vi "BeeperCAL2014.VI"(0 "offset":dbl=137.0, 1 "Init":bool=TRUE, 2 "sample rate":dbl=48000.0, 3 "number of samples":i32=512, 4 "Upper Cut-Off":dbl=4000.0, 5 "Lower Cut-Off":dbl=2000.0, 7 "error in":errorcluster, 19 "Serial":string) -> (10 "N Harmonics":i32, 12 "Harmonic Array":T1(array[cluster]), 13 "error out":errorcluster, 14 "PASS/FAIL 4":bool caption="PASS/FAIL", 15 "fundamental frequency":dbl format="%.2p", 16 "fundamental amplitude":dbl, 17 "fundamental dB output":dbl, 18 "THD":dbl format="%.2p")   [LabVIEW 2014]
uses:
  <vilib>/express/express analysis/Spectral/Block/exnSpectralBlock spectral measurements peak poly.vi
  <vilib>/express/express analysis/Spectral/Block/exnSpectralBlock spectral measurements peak WFM.vi
  <vilib>/measure/matone.llb/Extract Multiple Tone Information 1 Chan.vi
  <vilib>/measure/matone.llb/Harmonic Distortion Analyzer 1 Chan.vi
  <vilib>/express/express analysis/Spectral/XNode/ExpressSpectralMeasurementsBlockNode.xnode
  <vilib>/measure/NI_MAPro.lvlib
panel:
  out "Beeper Time Domain AC":waveform(dbl)(graph)={"t0"=timestamp(0.0010416666666666667 s since 1904-01-01), "dt"=2.0833333333333333e-05, "Y"=array[205 elements], "attributes"=variant("NI_ChannelName"=variant(string "Filtered (Extracted)"), "NI_ExpIsRelativeTime"=variant(bool TRUE), "NI_ExpStartTimeStamp"=variant(timestamp timestamp(3490807910.470092 s since 1904-01-01)), "NI_ExpTimeStamp"=variant(timestamp timestamp(3490807910.4711337 s since 1904-01-01)), "NI_ExpXDimension"=variant(string "t"), "NI_OriginalChannelName"=variant(string "Filtered"))}
  out "FFT Mask":dynamicdata(graph)=[{"t0"=timestamp(0 s since 1904-01-01), "dt"=160.53511884163183, "Y"=[0.01862930946391062, 0.031426642217661484, 0.028979598239673703, 0.024709926366084507, 0.012017232364681342, 0.011717656169097746, 0.011122701775221618, 0.001466420910336564, 0.007559244860713749, 0.009360343024873896, 0.003456556665288603, 0.0067897156296726074, 0.006203684074720098, 0.00631879509417875, 0.012993104805963341, 0.013327012696816912, 0.0356049653294887, 0.2818839469028935, 1.2722755465923246, 1.198586262791819, 0.2096225801168994, 0.03758360783596433, 0.010470687908423763, 0.0044974648911843005, 0.004067655995640319, 0.0012643427161311317, 0.0018238117756748699, 0.003084844757409455, 0.00168924041789103, 0.0034902948133270135, 0.0018217384819525847, 0.00188115142234715, 0.0013349862994453566, 0.0012364116957955678, 0.0009009915470407127, 0.0016168191099444537, 0.003914549671586599, 0.007639197093317019, 0.0025429875562595315, 0.0008863144299645895, 0.000625970666921518, 0.00012529417135776933, 0.00022916937706817103, 8.05943746999969e-05, 0.0002947428004910281, 0.0002087071302997354, 0.00040486818402033474, 0.0003375545596782854, 0.0002959939659886654, 0.0002699299152619309, 0.00013911678768285866, 4.346861415304848e-05, 0.0001340626371251187, 0.00016265618612929948, 0.0001476836700813654, 0.00039981352334013366, 0.00035508436857194415, 6.626140200756173e-05, 3.88995080941158e-05, 3.119123025937372e-05, 2.5285638387376754e-05, 4.886844544186635e-05, 7.271737186606323e-05, 5.3880406295179994e-05, 1.0072539300096652e-05, 2.3422235573147303e-05, 3.2314657446449763e-06, 1.6990206739975872e-05, 1.134108398471203e-05, 4.178417309496945e-06, 1.0252243489860926e-05, 9.766164633672498e-06, 1.3132869053438505e-05, 1.527288254858445e-05, 3.3272188602078897e-05, 1.2771336225145865e-05, 4.473167784884164e-06, 4.620966317927218e-06, 5.8214805857980874e-06, 2.379626005199326e-06, 2.9329660287990012e-06, 1.3631432808303542e-06, 3.4991665124997253e-06, 1.0655970567577459e-06, 4.419526022999793e-07, 2.1382029521115426e-06, 1.475862427158877e-07, 1.9584391227532084e-06, 2.0860245880026544e-06, 2.129493795041458e-06, 1.121334519682653e-06, 2.872638431024709e-06, 1.8550832235640507e-06, 1.4625248451505506e-06, 5.315345648632081e-07, 8.534708408493283e-07, 3.283129119564777e-07, 5.02807829864226e-07, 2.4382890249089887e-07, 6.188312885710458e-07, 5.081982604412368e-07, 2.1608286873766714e-07, 4.989348320620008e-07, 4.019887501348107e-07, 2.6797818414105616e-07, 4.4343144544713926e-07, 2.739673611594064e-07, 3.601606569482968e-07, 2.4474532583807605e-07, 2.836248881840115e-07, 3.176917348943672e-07, 2.1349864844518757e-07, 2.92082878448765e-07, 2.214756065002239e-07, 2.8606260405775217e-07, 1.8201583112405534e-07, 2.4372776748657747e-07, 2.028220893859686e-07, 2.0375064159335707e-07, 2.1300679020045898e-07, 1.7890992742712778e-07, 1.8547111735493437e-07, 1.7611449860683832e-07, 1.7875609596142585e-07, 1.6297443335424254e-07, 1.589828987944283e-07, 1.5841649477268463e-07, 1.456025867482396e-07, 1.4721535218519734e-07, 1.383699844195478e-07, 1.3710525723389903e-07, 1.305385615924326e-07, 1.2606070999131247e-07, 1.227773533123688e-07, 1.1920861575851639e-07, 1.1531047964591549e-07, 1.1224234459715743e-07, 1.0871712177752873e-07, 1.0589636424703531e-07, 1.031615300858949e-07, 1.0068840478885112e-07, 9.833545832303213e-08, 9.629379899415174e-08, 9.448219109599016e-08, 9.29052890739438e-08, 9.158747866699481e-08, 9.052317514966884e-08, 8.972112518164855e-08, 8.918448214399814e-08, 8.891552686030246e-08]}, {"t0"=timestamp(0 s since 1904-01-01), "dt"=160.53511884163183, "Y"=[nan, nan, nan, nan, nan, nan, nan, nan, nan, nan, nan, nan, nan, nan, nan, nan, nan, nan, nan, nan, nan, nan, nan, nan, nan, nan, nan, nan, nan, nan, nan, nan, nan, nan, nan, nan, nan, nan, nan, nan, nan, nan, nan, nan, nan, nan, nan, nan, nan, nan, nan, nan, nan, nan, nan, nan, nan, nan, nan, nan, nan, nan, nan, nan, nan, nan, nan, nan, nan, nan, nan, nan, nan, nan, nan, nan, nan, nan, nan, nan, nan, nan, nan, nan, nan, nan, nan, nan, nan, nan, nan, nan, nan, nan, nan, nan, nan, nan, nan, nan, nan, nan, nan, nan, nan, nan, nan, nan, nan, nan, nan, nan, nan, nan, nan, nan, nan, nan, nan, nan, nan, nan, nan, nan, nan, nan, nan, nan, nan, nan, nan, nan, nan, nan, nan, nan, nan, nan, nan, nan, nan, nan, nan, nan, nan, nan, nan, nan, nan, nan], "attributes"=variant("NI_ChannelName"=variant(string "Failures"))}, {"t0"=timestamp(0 s since 1904-01-01), "dt"=160.53511884163183, "Y"=[10.0, 10.0, 10.0, 0.05, 0.05, 0.05, 0.05, 0.05, 0.05, 0.05, 0.05, 0.05, 0.05, 0.05, 0.05, 0.05, 20.0, 20.0, 20.0, 20.0, 20.0, 20.0, 7.322726808155797, 0.05, 0.05, 0.05, 0.05, 0.05, 0.05, 0.05, 0.05, 0.05, 0.05, 0.05, 0.05, 0.05, 6.0, 6.0, 6.0, 6.0, 0.05, 0.05, 0.05, 0.05, 0.05, 0.05, 0.05, 0.05, 0.05, 0.05, 0.05, 0.05, 0.05, 0.05, 5.0, 5.0, 5.0, 5.0, 3.9404582897940448, 0.2, 0.2, 0.2, 0.2, 0.2, 0.2, 0.2, 0.2, 0.2, 0.2, 0.2, 0.2, 0.2, 0.2, 0.2, 0.2, 0.2, 0.2, 0.2, 0.2, 0.2, 0.2, 0.2, 0.2, 0.2, 0.2, 0.2, 0.2, 0.2, 0.2, 0.2, 0.2, 0.2, 0.2, 0.2, 0.2, 0.2, 0.2, 0.2, 0.2, 0.2, 0.2, 0.2, 0.2, 0.2, 0.2, 0.2, 0.2, 0.2, 0.2, 0.2, 0.2, 0.2, 0.2, 0.2, 0.2, 0.2, 0.2, 0.2, 0.2, 0.2, 0.2, 0.2, 0.2, 0.2, 0.2, 0.2, 0.2, 0.2, 0.2, 0.2, 0.2, 0.2, 0.2, 0.2, 0.2, 0.2, 0.2, 0.2, 0.2, 0.2, 0.2, 0.2, 0.2, 0.2, 0.2, 0.2, 0.2, 0.2, 0.2, 0.2], "attributes"=variant("NI_ChannelName"=variant(string "Upper Limit"))}, {"t0"=timestamp(0 s since 1904-01-01), "dt"=160.53511884163183, "Y"=[0.0, 0.0, 0.0, 0.0, 0.0, 0.0, 0.0, 0.0, 0.0, 0.0, 0.0, 0.0, 0.0, 0.0, 0.0, 0.0, 0.0, 0.0, 0.0, 0.0, 0.0, 0.0, 0.0, 0.0, 0.0, 0.0, 0.0, 0.0, 0.0, 0.0, 0.0, 0.0, 0.0, 0.0, 0.0, 0.0, 0.0, 0.0, 0.0, 0.0, 0.0, 0.0, 0.0, 0.0, 0.0, 0.0, 0.0, 0.0, 0.0, 0.0, 0.0, 0.0, 0.0, 0.0, 0.0, 0.0, 0.0, 0.0, 0.0, 0.0, 0.0, 0.0, 0.0, 0.0, 0.0, 0.0, 0.0, 0.0, 0.0, 0.0, 0.0, 0.0, 0.0, 0.0, 0.0, 0.0, 0.0, 0.0, 0.0, 0.0, 0.0, 0.0, 0.0, 0.0, 0.0, 0.0, 0.0, 0.0, 0.0, 0.0, 0.0, 0.0, 0.0, 0.0, 0.0, 0.0, 0.0, 0.0, 0.0, 0.0, 0.0, 0.0, 0.0, 0.0, 0.0, 0.0, 0.0, 0.0, 0.0, 0.0, 0.0, 0.0, 0.0, 0.0, 0.0, 0.0, 0.0, 0.0, 0.0, 0.0, 0.0, 0.0, 0.0, 0.0, 0.0, 0.0, 0.0, 0.0, 0.0, 0.0, 0.0, 0.0, 0.0, 0.0, 0.0, 0.0, 0.0, 0.0, 0.0, 0.0, 0.0, 0.0, 0.0, 0.0, 0.0, 0.0, 0.0, 0.0, 0.0, 0.0], "attributes"=variant("NI_ChannelName"=variant(string "Lower Limit"))}]
  out "number of cycles \nbefore sample acquisition":i32
  out "Beeper Time Domain":waveform(dbl)(graph)={"t0"=timestamp(3481896339.6964803 s since 1904-01-01), "dt"=2.0833333101715314e-05, "Y"=array[299 elements], "attributes"=variant("NI_ChannelName"=variant(string "Voltage_7 (Trigger)"), "NI_OriginalChannelName"=variant(string "Voltage_7"), "NI_UnitDescription"=variant(string "Volts"))}
  out "FFT Peak":cluster{"f0":dbl, "df":dbl, "magnitude":dbl[]}(graph)={"f0"=0.0, "df"=160.53511884163183, "magnitude"=[0.00013598036105044248, 0.00022939154903402542, 0.00021152991415820222, 0.0001803644260298139, 8.771702455971783e-05, 8.553033700071347e-05, 8.118760419869794e-05, 1.0703802265230393e-05, 5.517696978623174e-05, 6.8323671714408e-05, 2.5230340622544545e-05, 4.955996809980006e-05, 4.528236550890583e-05, 4.612259192831205e-05, 9.484018106542584e-05, 9.727746494026943e-05, 0.0002598902578794796, 0.0020575470576853537, 0.009286682821841785, 0.008748804837896489, 0.0015300918256707986, 0.0002743329039121484, 7.642837889360411e-05, 3.282821088455694e-05, 2.969091967620671e-05, 9.228778949862275e-06, 1.3312494712955255e-05, 2.2517115017587263e-05, 1.2330222028401678e-05, 2.5476604476839515e-05, 1.3297361182135654e-05, 1.3731032279906205e-05, 9.744425543396763e-06, 9.024902889018744e-06, 6.576580635333669e-06, 1.1801599342660246e-05, 2.8573355267055465e-05, 5.5760562724941746e-05, 1.856195296539804e-05, 6.469448393902113e-06, 4.569128955631518e-06, 9.145559953121849e-07, 1.6727691756800804e-06, 5.882801072992474e-07, 2.1514073028542195e-06, 1.5234097102170466e-06, 2.955242219126531e-06, 2.463901895461937e-06, 2.1605398977274845e-06, 1.970291352276868e-06, 1.0154510049843698e-06, 3.1728915440181375e-07, 9.785593950738592e-07, 1.1872714316007262e-06, 1.077982993294638e-06, 2.9183468856944063e-06, 2.5918567049047017e-06, 4.836598686683338e-07, 2.839380152855168e-07, 2.2767321357207097e-07, 1.8456670355749456e-07, 3.567039813274916e-07, 5.307837362486367e-07, 3.9328763719109487e-07, 7.352218467223834e-08, 1.7096522316165916e-07, 2.3587341201788147e-08, 1.2401610759106476e-07, 8.278163492490532e-08, 3.049939641968573e-08, 7.48338940865761e-08, 7.128587323848539e-08, 9.586035805429566e-08, 1.1148089451521497e-07, 2.4286269052612335e-07, 9.322143230033478e-08, 3.265085974368003e-08, 3.372968115275342e-08, 4.249255902042399e-08, 1.7369532884666614e-08, 2.1408511159116796e-08, 9.94995095496609e-09, 2.5541361405107483e-08, 7.778080706260918e-09, 3.225931403649484e-09, 1.560732081833243e-08, 1.077271844641516e-09, 1.4295176078490571e-08, 1.5226456846734706e-08, 1.5543750328769767e-08, 8.184923501333234e-09, 2.0968163730107363e-08, 1.3540753456671903e-08, 1.0675363833215697e-08, 3.879814342067212e-09, 6.229714166783418e-09, 2.396444612821005e-09, 3.6701301449943505e-09, 1.7797730108824734e-09, 4.5170167048981446e-09, 3.70947635358567e-09, 1.5772472170632637e-09, 3.6418600880438017e-09, 2.934224453538764e-09, 1.9560451397157385e-09, 3.236725879176199e-09, 1.9997617602876377e-09, 2.6289099047320936e-09, 1.7864622323947156e-09, 2.070254658277456e-09, 2.3189177729515854e-09, 1.5583842952203472e-09, 2.1319918134946352e-09, 1.616610266424992e-09, 2.088048204801111e-09, 1.3285827089347105e-09, 1.7790347991720982e-09, 1.4804532071968512e-09, 1.487230960535453e-09, 1.554794089054445e-09, 1.3059118790301297e-09, 1.3538037763133895e-09, 1.2855072891010097e-09, 1.304789021616247e-09, 1.189594404045566e-09, 1.1604591152877979e-09, 1.1563247793626615e-09, 1.0627926040017489e-09, 1.0745646144904915e-09, 1.0099998862740714e-09, 1.000768300977365e-09, 9.528362160031577e-10, 9.20151167819799e-10, 8.961850606742249e-10, 8.701358814490247e-10, 8.416823331818649e-10, 8.192871868405652e-10, 7.935556334126185e-10, 7.729661623871191e-10, 7.530038692401087e-10, 7.349518597726359e-10, 7.177770680513294e-10, 7.028744452127864e-10, 6.896510298977384e-10, 6.781407961601738e-10, 6.685217420948527e-10, 6.607531032822543e-10, 6.548987239536391e-10, 6.509816214890375e-10, 6.490184442357844e-10]}
  # "Trigger at 0.8"
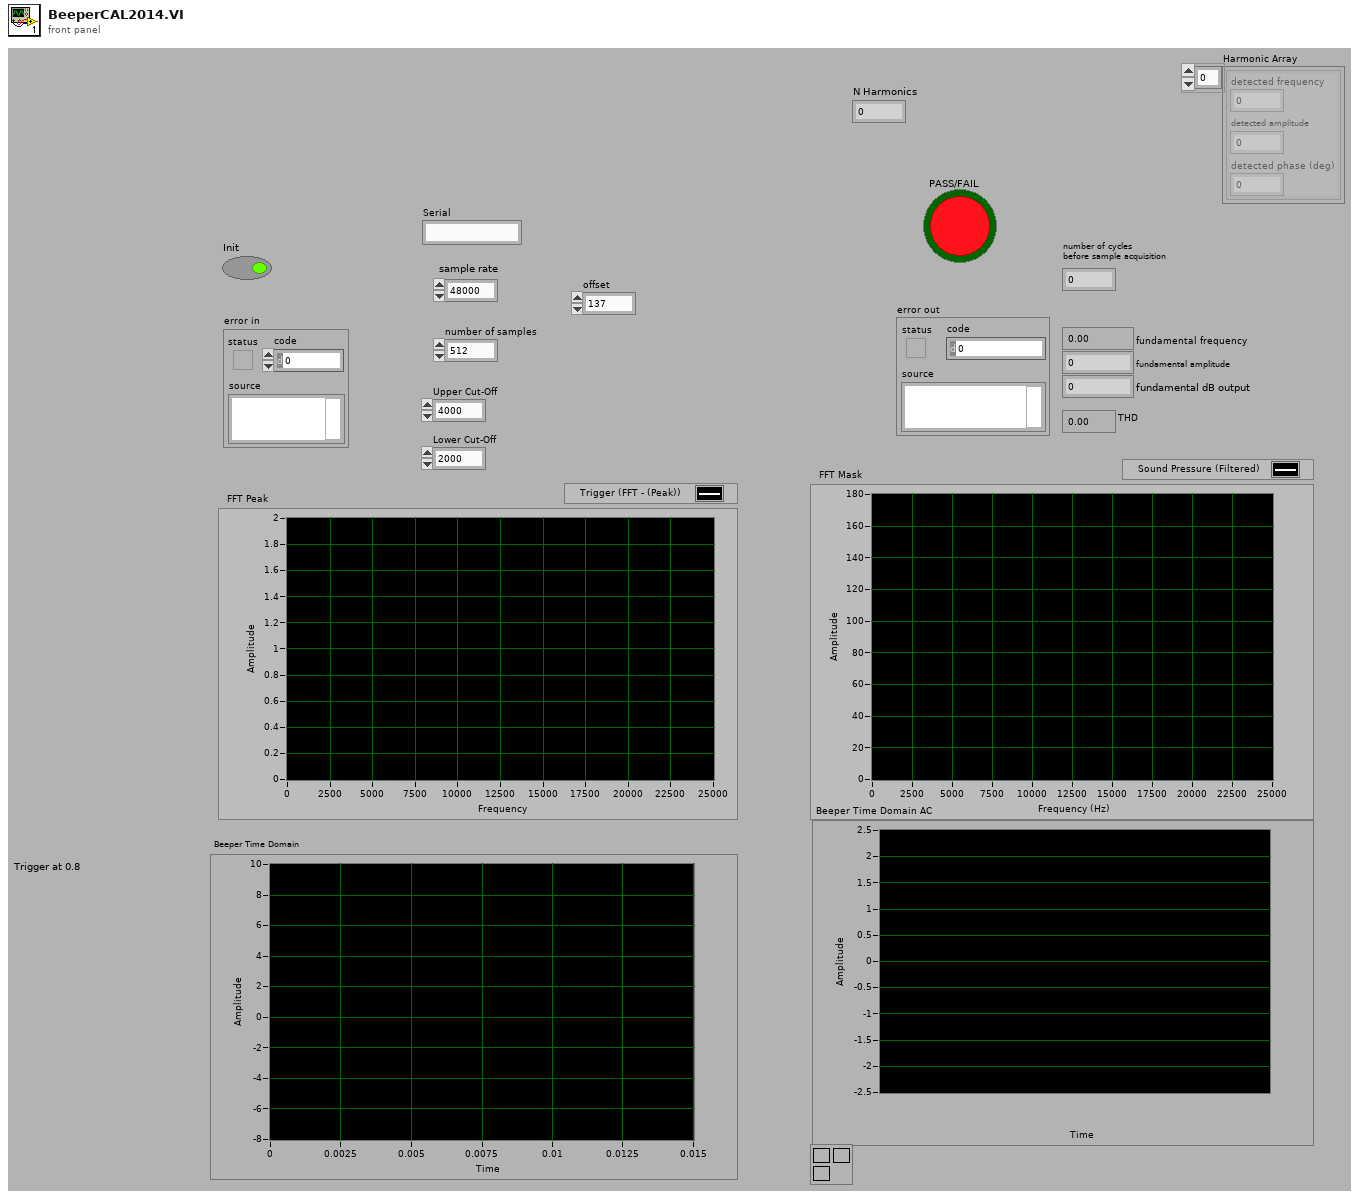
[diagram p1: front panel]
types:
  T1 = cluster{"detected frequency":dbl, "detected amplitude":dbl, "detected phase (deg)":dbl}[]
  T2 = cluster{"averaging mode":u16, "weighting mode":u16, "number of averages":u32}
  T3 = cluster{"dB On (F)":bool, "unwrap phase (F)":bool, "convert to degree (F)":bool}
  T4 = enum32{"none", "input signal", "detected signal", "residual signal"}
  T5 = cluster{"approx freq. (optional)":dbl, "search (+/- % of Fsampl.)":dbl}
  T6 = enum16{"none", "input signal", "fundamental signal", "residual signal", "harmonics only", "noise and spurs"}
  T7 = cluster{"detected frequency":dbl, "detected amplitude":dbl, "detected phase (deg)":dbl}
  T8 = cluster{"detected frequency":dbl, dbl, "detected phase (deg)":dbl}
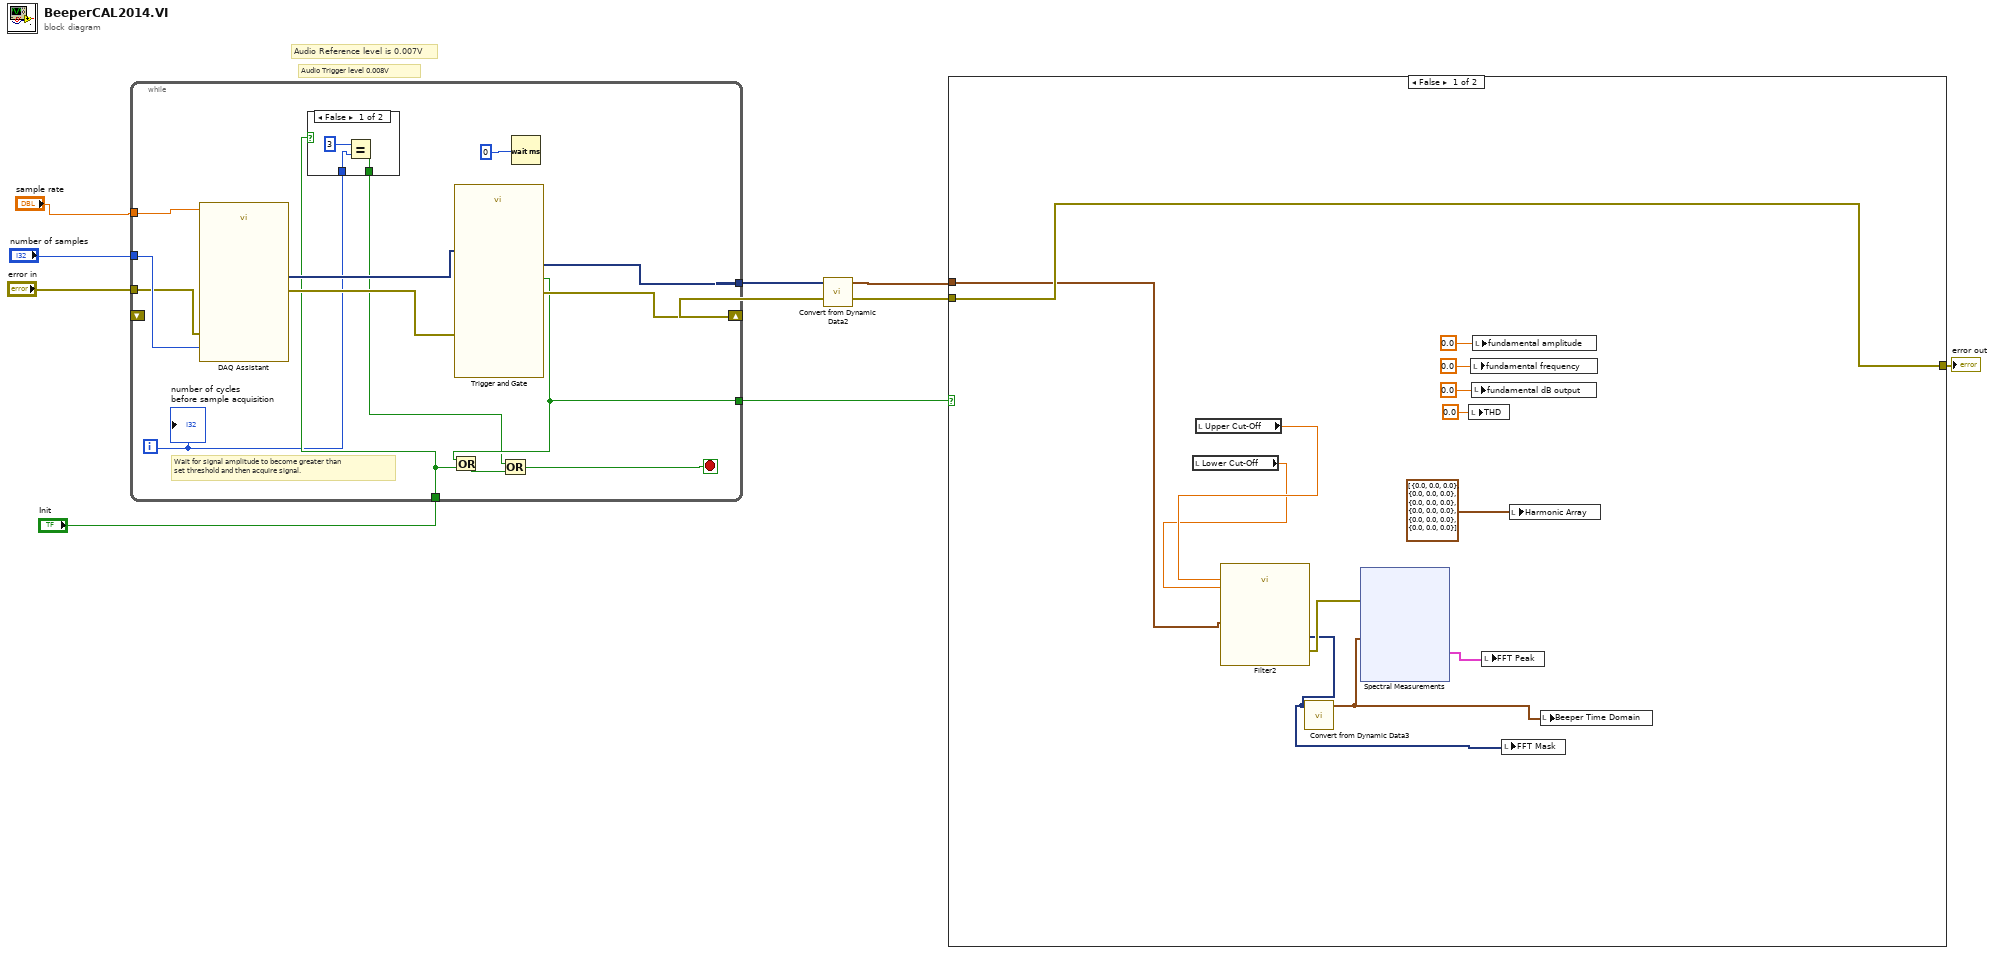
[diagram p0: block diagram]
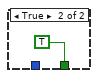
[diagram p2: hidden frame]
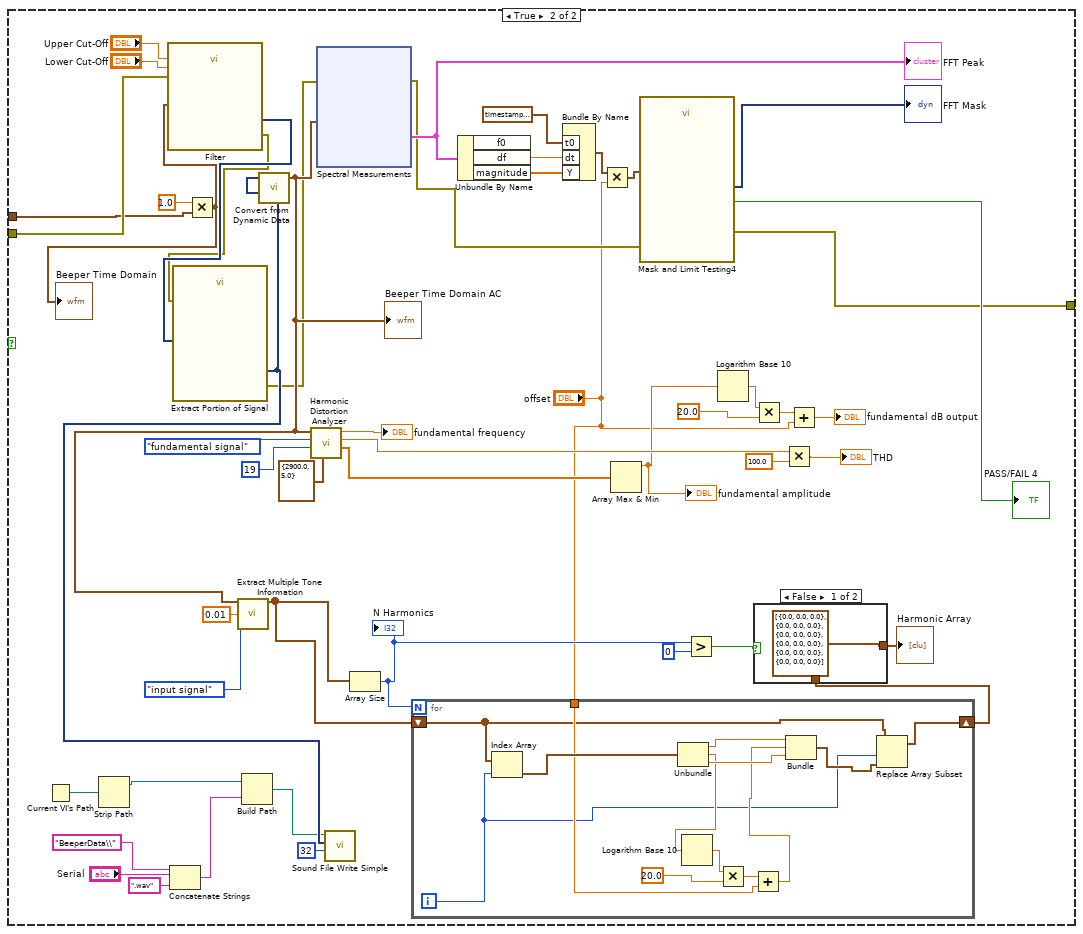
[diagram p3: hidden frame]
diagram:
  # "Audio Trigger level 0.008V"
  # "Audio Reference level is 0.007V"
  n1 = while {
    tunnel: [w15] -> w6
    shift-right: [w21] -> w5
    shift-left: _ -> [_]
    tunnel: [w23] -> w4
    tunnel: "sample rate" -> [w19]
    tunnel: "number of samples" -> [w18]
    tunnel: "error in" -> [w16]
    tunnel: "Init" -> [w12]
    i -> [w10]
    stop <- w13 stop-if-true
    # "Wait for signal amplitude to become greater than\nset threshold and then acquire signal."
    n2 = call "DAQ Assistant"("rate"=w19, "number of samples"=w18, "error in"=w16) -> ("data"=w20:dynamicdata, "error out"=w17:errorcluster)  [unwired: 13 in, 2 out]
    n3 = case shown="False" w12 {
      tunnel: w10 -> [w26 _]
      tunnel: [w24 TRUE] -> w11
      frame False {
        n4 = Equal?(x=3, y=w26) -> (x = y?=w24:bool)
      }
      frame True {
      }
    }
    n5 = call "Trigger and Gate"("error in (no error)"=w17, "Signals"=w20) -> ("error out"=w21:errorcluster, "Triggered Signals"=w23:dynamicdata, "Data Available"=w15:bool)  [unwired: 6 in, 1 out]
    n6 = Or(x=w15, y=w12) -> (x .or. y?=w14:bool)
    n7 = Or(x=w11, y=w14) -> (x .or. y?=w13:bool)
    n8 = Wait (ms)(milliseconds to wait=u32 0) -> ()  [unwired: 1 out]
    "number of cycles \nbefore sample acquisition" <- w10
  }
  n9 = call "Convert from Dynamic Data2"("Dynamic Data Type"=w4) -> ("Waveform"=w7:waveform(dbl))  [unwired: 3 in]
  n10 = case shown="False" w6 {
    tunnel: w7 -> [w33 w97]
    tunnel: w5 -> [w40 w98]
    tunnel: [w40 w99] -> w2
    frame False {
      n11 = local read "Lower Cut-Off"() -> (w31:dbl)
      n12 = local read "Upper Cut-Off"() -> (w32:dbl)
      n13 = call "Filter2"("Lower Cut-Off"=w31, "Upper Cut-Off"=w32, "Signal"=w33) -> ("error out"=w34:errorcluster, "Filtered Signal"=w29:dynamicdata)  [unwired: 7 in]
      n14 = call "Convert from Dynamic Data3"("Dynamic Data Type"=w29) -> ("Waveform"=w30:waveform(dbl))  [unwired: 3 in]
      n15 = xnode "Spectral Measurements"("Signals"=w30, "error in (no error)"=w34) -> ("FFT - (Peak)"=w28:cluster{"f0":dbl, "df":dbl, "magnitude":dbl[]})  [unwired: 2 out]
      n16 = local write "THD"(0.0 ("THD")) -> ()
      n17 = local write "fundamental frequency"(0.0 ("fundamental frequency")) -> ()
      n18 = local write "fundamental dB output"(0.0 ("fundamental dB output")) -> ()
      n19 = local write "fundamental amplitude"(0.0 ("fundamental amplitude")) -> ()
      n20 = local write "FFT Peak"(w28) -> ()
      n21 = local write "FFT Mask"(w29) -> ()
      n22 = local write "Harmonic Array"(T1 [{"detected frequency"=0.0, "detected amplitude"=0.0, "detected phase (deg)"=0.0}, {"detected frequency"=0.0, "detected amplitude"=0.0, "detected phase (deg)"=0.0}, {"detected frequency"=0.0, "detected amplitude"=0.0, "detected phase (deg)"=0.0}, {"detected frequency"=0.0, "detected amplitude"=0.0, "detected phase (deg)"=0.0}, {"detected frequency"=0.0, "detected amplitude"=0.0, "detected phase (deg)"=0.0}, {"detected frequency"=0.0, "detected amplitude"=0.0, "detected phase (deg)"=0.0}] ("multiple tone information")) -> ()
      n23 = local write "Beeper Time Domain"(w30) -> ()
    }
    frame True {
      n24 = Current VI's Path() -> (path=w56:path)
      n25 = Strip Path(path=w56) -> (stripped path=w55:path)  [unwired: 1 out]
      n26 = Concatenate Strings("BeeperData\\" ("string"), "Serial", ".wav" ("string")) -> (w60:string)
      n27 = Multiply(x=1.0, y=w97) -> (x*y=w95:waveform(dbl))
      "Beeper Time Domain" <- w95
      n28 = call "Filter"("error in (no error)"=w98, "Lower Cut-Off"="Lower Cut-Off", "Upper Cut-Off"="Upper Cut-Off", "Signal"=w95) -> ("error out"=w51:errorcluster, "Filtered Signal"=w63:dynamicdata)  [unwired: 6 in]
      n29 = call "Extract Portion of Signal"("error in (no error)"=w51, "Signals"=w63) -> ("error out"=w52:errorcluster, "Section"=w61:dynamicdata)  [unwired: 8 in]
      n30 = Build Path(base path=w55, name or relative path=w60) -> (appended path=w54:path)
      n31 = call "Convert from Dynamic Data"("Dynamic Data Type"=w61) -> ("Waveform"=w53:waveform(dbl))  [unwired: 3 in]
      "Beeper Time Domain AC" <- w53
      n32 = call-poly <vilib>:"Extract Multiple Tone Information.vi"("time signal in"=w53, "export mode"=T4."input signal", "threshold"=0.01) -> ("multiple tone information"=w71:T1)  [unwired: 10 in, 2 out]
      n33 = call-poly <vilib>:"Harmonic Distortion Analyzer.vi"("advanced search"=T5 {"approx freq. (optional)"=2900.0, "search (+/- % of Fsampl.)"=5.0}, "highest harmonic"=19, "export mode"=T6."fundamental signal" ("export signals"), "signal in"=w53) -> ("components level"=w88:dbl[], "THD"=w78:dbl, "detected fundamental frequency"=→"fundamental frequency":dbl)  [unwired: 2 in, 3 out]
      n34 = xnode "Spectral Measurements"("Signals"=w53, "error in (no error)"=w52) -> ("FFT - (Peak)"=w94:cluster{"f0":dbl, "df":dbl, "magnitude":dbl[]}, "error out"=w74:errorcluster)  [unwired: 1 out]
      "FFT Peak" <- w94
      n35 = call <vilib>:"Sound File Write Simple.vi"("bits per sample"=32, "data"=w61, "path"=w54) -> ()  [unwired: 7 in, 2 out]
      n36 = Array Size(array=w71) -> (size(s)=w70:i32)
      "N Harmonics" <- w70
      n37 = for {
        N: w70 -> [_]
        tunnel: "offset" -> [w107]
        shift-right: [w105] -> w67
        shift-left: w71 -> [w104]
        i -> [w106]
        n38 = Index Array(array=w104, index=w106) -> (element=w116:T7)
        n39 = Unbundle(w116) -> ("detected frequency"=w115:dbl, "detected amplitude"=w109:dbl, "detected phase (deg)"=w114:dbl)
        n40 = Logarithm Base 10(1:w109) -> (0:w112:dbl)
        n41 = Multiply(x=w112, y=20.0) -> (x*y=w110:dbl)
        n42 = Add(x=w110, y=w107) -> (x+y=w108:dbl)
        n43 = Bundle("detected frequency"=w115, w108, "detected phase (deg)"=w114) -> (w113:T8)  [unwired: 1 in]
        n44 = Replace Array Subset(array=w104, new element=w113, index=w106) -> (w105:T1)
      }
      n45 = Unbundle By Name(w94) -> ("df"=w93:dbl, "magnitude"=w92:dbl[])  [unwired: 1 out]
      n46 = Bundle By Name("t0"=timestamp(0 s since 1904-01-01), "dt"=w93, "Y"=w92) -> (w75:waveform(dbl))  [unwired: 1 in]
      n47 = Multiply(x=w75, y="offset") -> (x*y=w76:waveform(dbl))
      n48 = Array Max & Min(array=w88) -> (max value=w77:dbl)  [unwired: 3 out]
      "fundamental amplitude" <- w77
      n49 = call "Mask and Limit Testing4"("error in"=w74, "Signals"=w76) -> ("error out"=w99:errorcluster, "Passed"=→"PASS/FAIL 4":bool, "Tested Signals"=→"FFT Mask":dynamicdata)  [unwired: 6 in, 1 out]
      n50 = Greater?(x=w70, y=0) -> (0:w68:bool)
      n51 = Logarithm Base 10(1:w77) -> (0:w87:dbl)
      n52 = Multiply(x=w87, y=20.0) -> (x*y=w85:dbl)
      n53 = case shown="False" w68 {
        tunnel: w67 -> [_ w103]
        tunnel: [T1 [{"detected frequency"=0.0, "detected amplitude"=0.0, "detected phase (deg)"=0.0}, {"detected frequency"=0.0, "detected amplitude"=0.0, "detected phase (deg)"=0.0}, {"detected frequency"=0.0, "detected amplitude"=0.0, "detected phase (deg)"=0.0}, {"detected frequency"=0.0, "detected amplitude"=0.0, "detected phase (deg)"=0.0}, {"detected frequency"=0.0, "detected amplitude"=0.0, "detected phase (deg)"=0.0}, {"detected frequency"=0.0, "detected amplitude"=0.0, "detected phase (deg)"=0.0}] ("multiple tone information") w103] -> w64
        frame False {
        }
        frame True {
        }
      }
      "Harmonic Array" <- w64
      n54 = Multiply(x=w78, y=100.0) -> (x*y=→"THD":dbl)
      n55 = Add(x=w85, y="offset") -> (x+y=→"fundamental dB output":dbl)
    }
  }
  "error out" <- w2
